vi "Main_014.vi"() -> ()   [LabVIEW 2018]
panel:
  out "Correct results":i16
  out "Wrongly classified as:\n square        triangle      circle     unclassified":dbl[](array[numeric])
  out "selected path":path[](array[path])
  out "Total wrong results":i16
  out "Results":string[](array[string])
  out "Template images":picture[](array[picture])
  in  "Open results":bool
  out "Correct?":bool[](array[boolean])
  out "dissimilarity values":dbl[](array[numeric])
  in  "Restart":bool
  in  "Start?":bool
  in  "Change files?":bool
  in  "stop":bool
  out "It's a":string
  in  "Decoder Parameters":T1
  in  "Encoder parameters":T2
  out "What's this?":picture
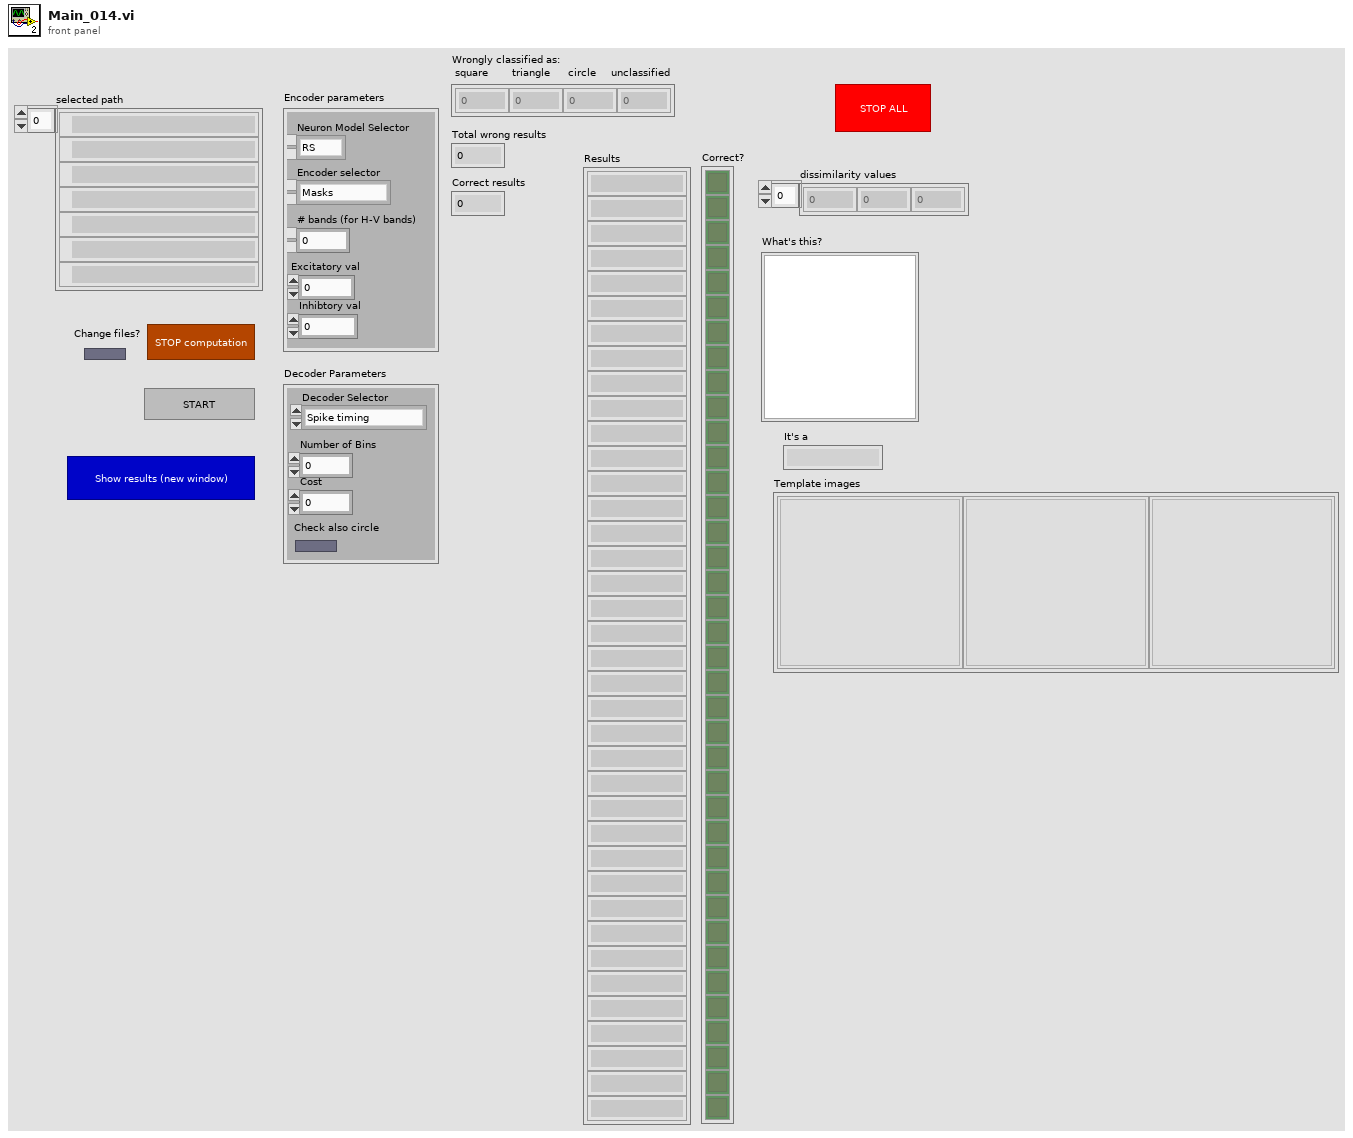
[diagram p1: front panel]
types:
  T1 = cluster{"Decoder Selector":enum16{"Spike timing", "Spike counting", "Victor Purpura"}, "Number of Bins":i32, "Cost":dbl, "Check also circle":bool}
  T2 = cluster{"Encoder selector":enum16{"Masks", "H-V bands", "Simple reading"}, "# bands (for H-V bands)":i32, "Excitatory val":dbl, "Inhibtory val":dbl, "Neuron Model Selector":enum16{"RS", "LTS", "RZ", "TC2", "TC1", "FS", "CH", "IB"}}
  T3 = cluster{"total duration":i32, "spike indexes":i32[]}
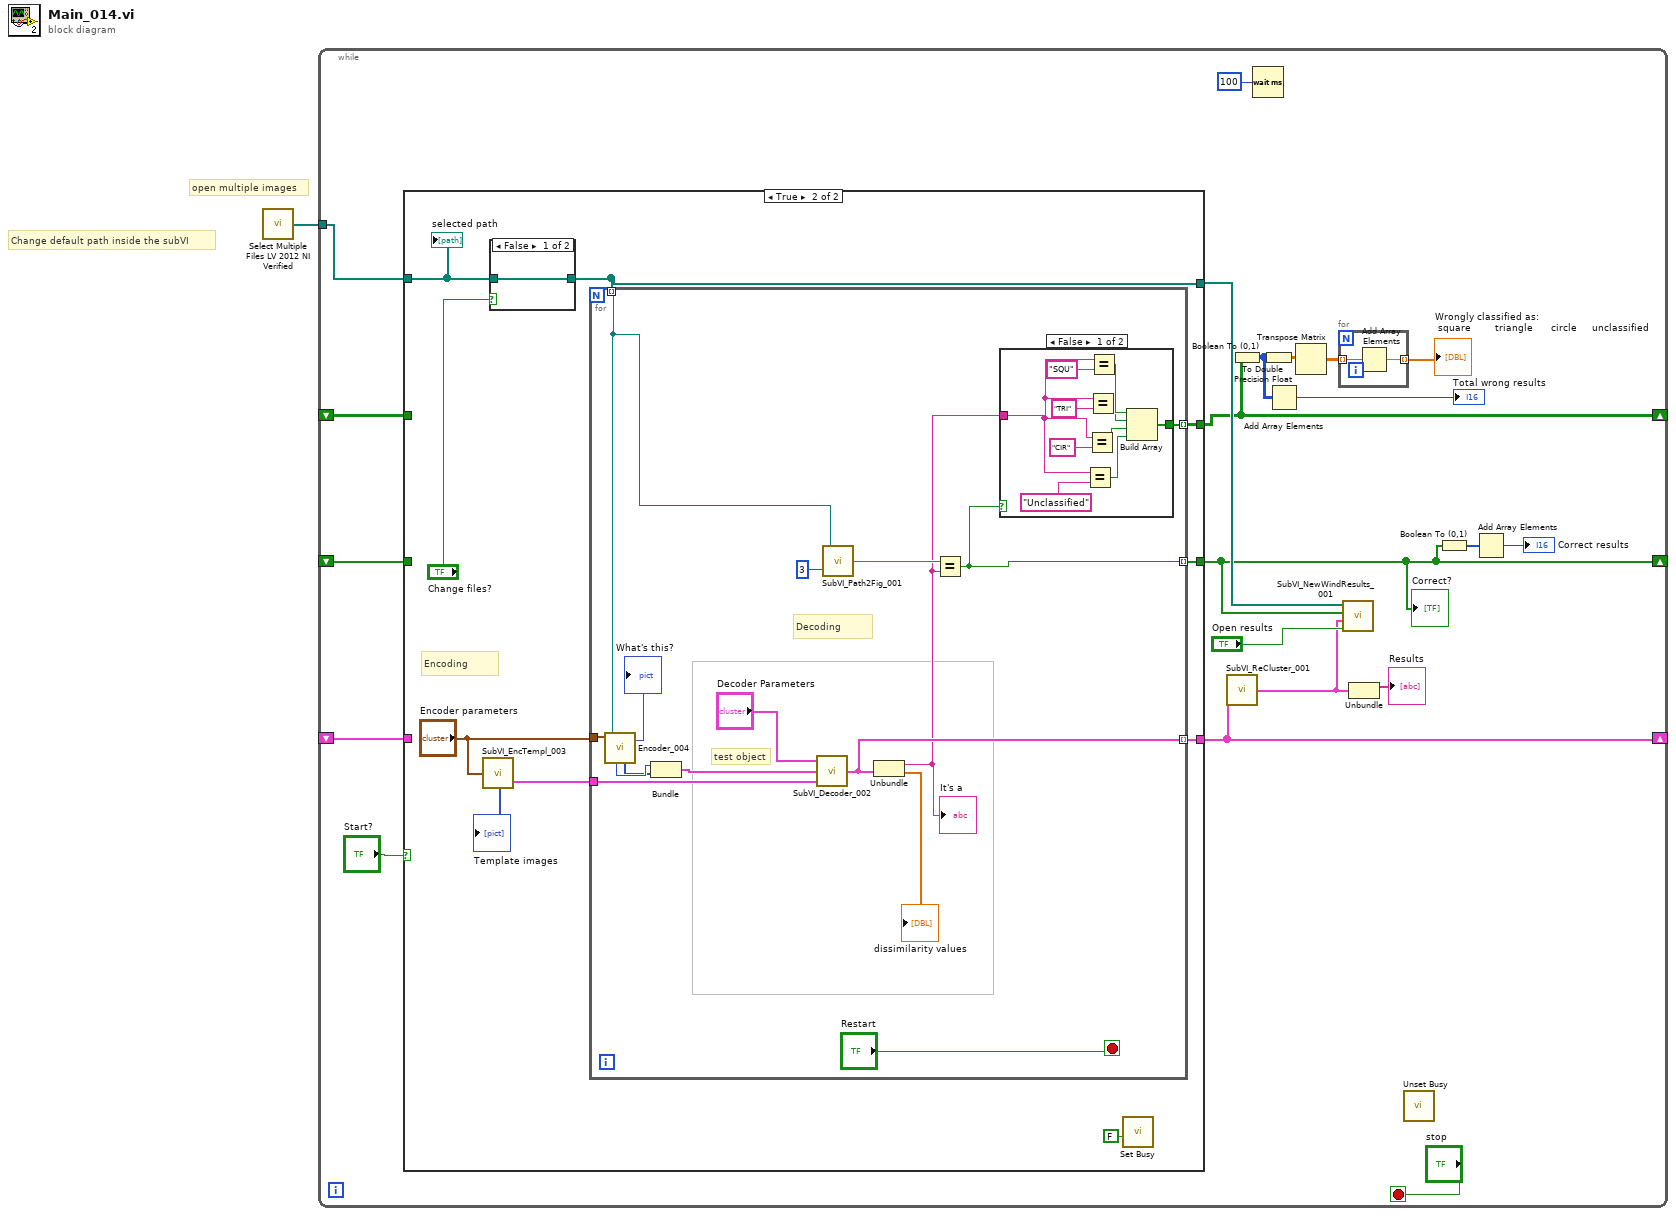
[diagram p0: block diagram]
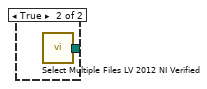
[diagram p3: hidden frame]
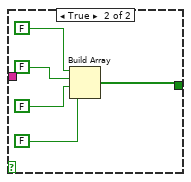
[diagram p4: hidden frame]
diagram:
  # "Change default path inside the subVI"
  # "open multiple images"
  n1 = call "Select Multiple Files LV 2012 NI Verified.vi"() -> ("selected path"=w1:path[])
  n2 = while {
    tunnel: w1 -> [w12]
    shift-right: [w4] -> _
    shift-left: _ -> [w20]
    shift-right: [w14] -> _
    shift-left: _ -> [w18]
    shift-right: [w10] -> _
    shift-left: _ -> [w11]
    stop <- "stop" stop-if-true
    n3 = case shown="True" "Start?" {
      tunnel: w12 -> [w27 w36]
      tunnel: [w28 w35] -> w4
      tunnel: w20 -> [w28 _]
      tunnel: [w27 w34] -> w17
      tunnel: [w26 w31] -> w14
      tunnel: w18 -> [w26 _]
      tunnel: [w25 w29] -> w10
      tunnel: w11 -> [w25 _]
      frame False {
      }
      frame True {
        # "Encoding"
        n4 = call "SubVI_EncTempl_003.vi"("Encoder parameters"="Encoder parameters") -> ("Template images"=→"Template images":picture[], "Cluster templates"=w33:cluster{i32[], i32[][]})
        n5 = case shown="False" "Change files?" {
          tunnel: [w39 w40] -> w34
          tunnel: w36 -> [w39 _]
          frame False {
          }
          frame True {
            n6 = call "Select Multiple Files LV 2012 NI Verified.vi"() -> ("selected path"=w40:path[])
          }
        }
        n7 = for {
          tunnel: "Encoder parameters" -> [w54]
          tunnel: w34 -> [w42] mode=indexing
          tunnel: [w47] -> w35 mode=indexing
          tunnel: w33 -> [w51]
          tunnel: [w49] -> w31 mode=indexing
          tunnel: [w41] -> w29 mode=indexing
          stop <- "Restart" stop-if-true
          # "test object"
          # "Decoding"
          n8 = call "Encoder_004.vi"("Image Path"=w42, "Encoder parameters"=w54) -> ("spike indexes"=w44:i32[], "total duration"=w45:i32, "Picture"=→"What's this?":picture)  [unwired: 4 in, 3 out]
          n9 = Bundle("total duration"=w45, "spike indexes"=w44) -> (w43:T3)  [unwired: 1 in]
          n10 = call "SubVI_Decoder_002.vi"("Cluster templates"=w51, "Object IMG Cluster"=w43, "Decoder Parameters"="Decoder Parameters") -> ("Results, dissimilarity, pixs"=w49:cluster{"Result":string, "Dissimilarity":dbl[]})
          n11 = call "SubVI_Path2Fig_001.vi"("length (rest)"=3, "Path"=w42) -> ("FIG"=w52:string)
          n12 = Unbundle(w49) -> ("Result"=w46:string, "Dissimilarity"=→"dissimilarity values":dbl[])
          "It's a" <- w46
          n13 = Equal?(x=w52, y=w46) -> (x = y?=w47:bool)
          n14 = case shown="False" w47 {
            tunnel: w46 -> [w63 _]
            tunnel: [w57 w67] -> w41
            frame False {
              n15 = Equal?(x=w63, y="Unclassified") -> (x = y?=w58:bool)
              n16 = Equal?(x=w63, y="CIR") -> (x = y?=w59:bool)
              n17 = Equal?(x=w63, y="TRI") -> (x = y?=w60:bool)
              n18 = Equal?(x=w63, y="SQU") -> (x = y?=w61:bool)
              n19 = Build Array(w61, w60, w59, w58) -> (w57:bool[])
            }
            frame True {
              n20 = Build Array(FALSE, FALSE, FALSE, FALSE) -> (w67:bool[])
            }
          }
        }
        n21 = call <vilib>:"Set Busy.vi"("disable click? (T)"=FALSE) -> ()  [unwired: 9 in, 2 out]
        "selected path" <- w36
      }
    }
    "Correct?" <- w4
    n22 = call "SubVI_ReCluster_001.vi"("Array"=w14) -> ("output cluster"=w13:cluster{string[], "Dissimilarity":dbl[][]})
    n23 = Boolean To (0,1)(Boolean=w10) -> (0, 1=w6:i16[][])
    n24 = Wait (ms)(milliseconds to wait=u32 100) -> ()  [unwired: 1 out]
    n25 = To Double Precision Float(number=w6) -> (double precision float=w7:dbl[][])
    n26 = Add Array Elements(numeric array=w6) -> (sum=→"Total wrong results":i16)
    n27 = Transpose Matrix(1:w7) -> (0:w9:dbl[][])
    n28 = for {
      tunnel: w9 -> [w24] mode=indexing
      tunnel: [w23] -> w8 mode=indexing
      n29 = Add Array Elements(numeric array=w24) -> (sum=w23:dbl)
    }
    "Wrongly classified as:\n square        triangle      circle     unclassified" <- w8
    n30 = call "SubVI_NewWindResults_001.vi"("Open results in another window"="Open results", "Results and dissimilarity"=w13, "Correct?"=w4, "paths"=w17) -> ()
    n31 = Unbundle(w13) -> (→"Results":string[])  [unwired: 1 out]
    n32 = call <vilib>:"Unset Busy.vi"() -> ()  [unwired: 11 in, 1 out]
    n33 = Boolean To (0,1)(Boolean=w4) -> (0, 1=w3:i16[])
    n34 = Add Array Elements(numeric array=w3) -> (sum=→"Correct results":i16)
  }
